vi "PubPlot.vi"() -> ()   [LabVIEW 2024]
uses:
  <vilib>/Utility/miscctls.llb/LVFontTypeDef.ctl
  <vilib>/Utility/miscctls.llb/LVBoundsTypeDef.ctl
panel:
  out "Plot Area:Size":T1
  in  "Axes":T3
  in  "FRF":cluster{"x0":dbl, "df":dbl, dbl[]}[](graph)
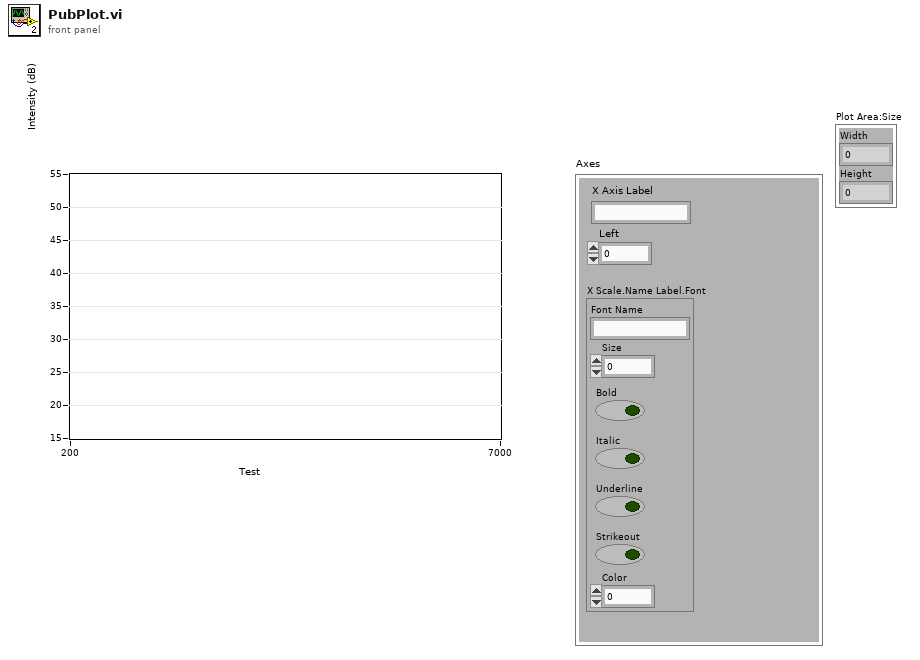
[diagram p1: front panel]
types:
  T1 = typedef "LVBoundsTypeDef.ctl" = cluster{"Width":u32, "Height":u32}
  T2 = typedef "LVFontTypeDef.ctl" = cluster{"Font Name":string, "Size":u16, "Bold":bool, "Italic":bool, "Underline":bool, "Strikeout":bool, "Color":u32}
  T3 = cluster{"X Axis Label":string, "Left":i32, "X Scale.Name Label.Font":T2}
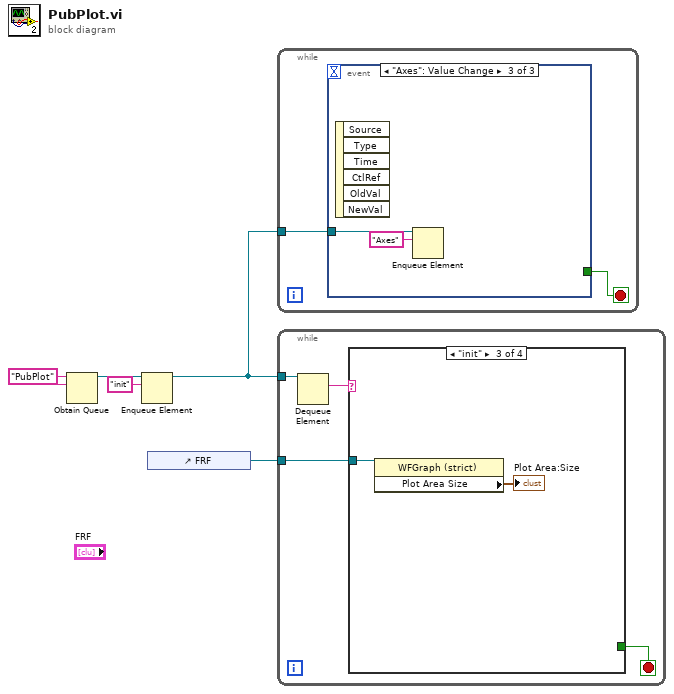
[diagram p0: block diagram]
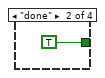
[diagram p3: hidden frame]
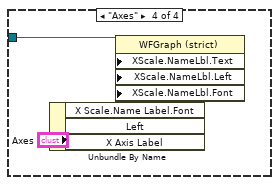
[diagram p4: hidden frame]
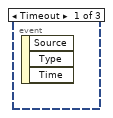
[diagram p5: hidden frame]
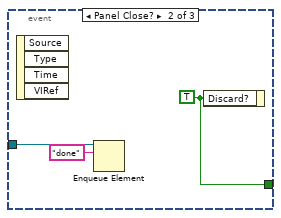
[diagram p6: hidden frame]
diagram:
  w4 = "PubPlot" ("name (unnamed)")
  n1 = Obtain Queue(name (unnamed)=w4, element data type=w4) -> (queue out=w5:refnum<queue>)  [unwired: 3 in, 2 out]
  n2 = Enqueue Element(queue=w5, element="init") -> (queue out=w2:refnum<queue>)  [unwired: 2 in, 2 out]
  n3 = control-ref of="FRF"() -> (w1:refnum<vi>)
  n4 = while {
    tunnel: w2 -> [w6]
    stop <- w7 stop-if-true
    n5 = event shown="[2] \"Axes\": Value Change" {
      selector: _ -> [_ _ _]
      dyn-events: _ -> [_ _ _]
      timeout: _ -> [_ _ _]
      tunnel: [_ w10 _] -> w7
      tunnel: w6 -> [_ w8 w11]
      event Timeout {
        n6 = event-data() -> ()  [unwired: 1 in, 3 out]
      }
      event Panel Close? {
        w10 = TRUE ("Discard?")
        n7 = event-data() -> ()  [unwired: 1 in, 4 out]
        n8 = Enqueue Element(queue=w8, element="done") -> ()  [unwired: 2 in, 3 out]
        n9 = event-data("Discard?"=w10) -> ()  [unwired: 1 in, 1 out]
      }
      event "Axes": Value Change {
        n10 = event-data() -> ()  [unwired: 1 in, 6 out]
        n11 = Enqueue Element(queue=w11, element="Axes") -> ()  [unwired: 2 in, 3 out]
      }
    }
  }
  n12 = while {
    tunnel: w2 -> [w16]
    tunnel: w1 -> [w13]
    stop <- w14 stop-if-true
    n13 = Dequeue Element(queue=w16) -> (element=w15:string)  [unwired: 2 in, 3 out]
    n14 = case shown="\"init\"" w15 {
      tunnel: [_ TRUE _ _] -> w14
      tunnel: w13 -> [_ _ w19 w23]
      frame Default {
      }
      frame "done" {
      }
      frame "init" {
        n15 = property class="WFGraph (strict)"(reference=w19) -> ("Plot Area Size"=→"Plot Area:Size":T1)  [unwired: 1 in, 2 out]
      }
      frame "Axes" {
        n16 = Unbundle By Name("Axes") -> ("X Scale.Name Label.Font"=w20:T2, "Left"=w21:i32, "X Axis Label"=w22:string)
        n17 = property class="WFGraph (strict)"(reference=w23, "XScale.NameLbl.Text"=w22, "XScale.NameLbl.Left"=w21, "XScale.NameLbl.Font"=w20) -> ()  [unwired: 1 in, 2 out]
      }
    }
  }
